vi "RL.vi"() -> ()   [LabVIEW 2019]
uses:
  <vilib>/Platform/TimedLoop/XDataNode/timing_clust.ctl
  <vilib>/Platform/TimedLoop/XDataNode/nitl_modes.ctl
  <vilib>/Platform/TimedLoop/XDataNode/wakeup.ctl
  <vilib>/Simulation/Shared/_Datatypes/SIM SISO Transfer Function.ctl
  <vilib>/myRIO/Instrument Drivers/Onboard IO/AI/typedefs/AI Reference.ctl
  <vilib>/myRIO/Common/Instrument Driver Framework/Utilities/typedefs/myRIO Generic Hardware Reference.ctl
  <vilib>/myRIO/Common/Instrument Driver Framework/Utilities/typedefs/Hardware Version Enum.ctl
  <vilib>/myRIO/Common/Instrument Driver Framework/Utilities/typedefs/myRIO v1.0 Reference.ctl
  <vilib>/myRIO/Common/Instrument Driver Framework/Utilities/typedefs/Generic FPGA Reference.ctl
  <vilib>/myRIO/Common/Instrument Driver Framework/myRIO v1.0/AI/typedefs/AI Channels List.ctl
  <vilib>/myRIO/Common/Instrument Driver Framework/myRIO v1.0/AI/typedefs/AI Channels Enum.ctl
  <vilib>/myRIO/Common/Instrument Driver Framework/Utilities/typedefs/Analog Scaling Constants List.ctl
  <vilib>/myRIO/Common/Instrument Driver Framework/Utilities/typedefs/Analog Scaling Constants.ctl
  <vilib>/userDefined/High Color/nirio_resource_hc.ctl
  <vilib>/Simulation/Shared/_Datatypes/SIM MIMO State Space.ctl
  <vilib>/myRIO/Instrument Drivers/Onboard IO/AO/typedefs/AO Reference.ctl
  <vilib>/myRIO/Common/Instrument Driver Framework/myRIO v1.0/AO/typedefs/AO Channels List.ctl
  <vilib>/myRIO/Common/Instrument Driver Framework/myRIO v1.0/AO/typedefs/AO Channels Enum.ctl
  <vilib>/myRIO/Common/Instrument Driver Framework/Utilities/vis/Is FPGA Ref Available.vi
  <vilib>/myRIO/Common/Instrument Driver Framework/myRIO v1.0/AI/vis/myRIO v1.1 Open AI.vi
  <vilib>/myRIO/Instrument Drivers/Onboard IO/AI/vis/Read.vi
  <vilib>/Simulation/DiscreteLinear/Implementation/NILVSim Discrete Transfer Function Direct.llb/SIM Discrete Transfer Function Diagram (SISO).vi
  <vilib>/Simulation/DiscreteLinear/Implementation/NILVSim Discrete State Space Direct.llb/SIM Discrete State Space Direct Diagram (SISO).vi
  <vilib>/myRIO/Common/Instrument Driver Framework/myRIO v1.0/AO/vis/myRIO v1.1 Open AO.vi
  <vilib>/myRIO/Instrument Drivers/Onboard IO/AO/vis/Write.vi
  <vilib>/myRIO/Common/Instrument Driver Framework/Utilities/vis/Validate Channels.vi
  <vilib>/myRIO/Common/Instrument Driver Framework/myRIO v1.0/AI/vis/myRIO v1.0 Reserve AI.vi
  <vilib>/Simulation/ContinuousLinear/Implementation/Shared/SIM Transfer Function Support.llb/SIM TransferFunction Normalize to Buffer.vi
  <vilib>/Simulation/DiscreteLinear/Implementation/Shared/SIM Init Discrete States.vi
  <vilib>/Simulation/DiscreteLinear/Implementation/NILVSim Discrete Transfer Function Direct.llb/SIM Transfer Function Direct core (SISO).vi
  <vilib>/Simulation/DiscreteLinear/Implementation/NILVSim Discrete State Space Direct.llb/NILVSim Discrete State Space Direct Diagram Core (SISO).vi
  <vilib>/myRIO/Common/Instrument Driver Framework/myRIO v1.0/AO/vis/myRIO v1.0 Reserve AO.vi
  <vilib>/myRIO/Common/Instrument Driver Framework/myRIO v1.0/AI/vis/myRIO v1.0 Build MUX Configuration AI.vi
  <vilib>/myRIO/Common/Instrument Driver Framework/myRIO v1.0/Resource Manager/vis/myRIO v1.0 Reserve Channel List.vi
  <vilib>/Simulation/ContinuousLinear/Implementation/Shared/SIM Transfer Function Support.llb/SIM TransferFunction Normalize.vi
  <vilib>/myRIO/Common/Instrument Driver Framework/myRIO v1.0/AO/vis/myRIO v1.0 Build MUX Configuration AO.vi
  <vilib>/myRIO/Common/Instrument Driver Framework/myRIO v1.0/Resource Manager/vis/myRIO v1.0 Reserve Channel.vi
  <vilib>/myRIO/Common/Instrument Driver Framework/myRIO v1.0/Resource Manager/vis/myRIO v1.0 Unreserve Channel.vi
  <vilib>/Simulation/Implementation/Shared/SIM Polynomials.llb/SIM Remove Zero Coefficients (DBL).vi
  <vilib>/myRIO/Common/Instrument Driver Framework/myRIO v1.0/Resource Manager/vis/myRIO v1.0 Build Mutex Name.vi
  <vilib>/Simulation/Implementation/Shared/SIM Polynomials.llb/SIM Divide Polynomials (DBL).vi
  <vilib>/Simulation/Implementation/Shared/SIM BuildSimErr.vi
  <vilib>/Utility/VariantDataType/GetNumericInfo.vi
  <vilib>/Utility/error.llb/Error Cluster From Error Code.vi
  <vilib>/myRIO/Common/Instrument Driver Framework/myRIO v1.0/myRIO v1.1 Open.vi
  <vilib>/myRIO/Common/Instrument Driver Framework/myRIO v1.0/AI/vis/myRIO v1.0 Get Scaling Constants AI.vi
  <vilib>/myRIO/Common/Instrument Driver Framework/Utilities/vis/IO Manager.vi
  <vilib>/myRIO/Common/Instrument Driver Framework/Utilities/vis/Configuration Manager.vi
  <vilib>/myRIO/Common/Instrument Driver Framework/myRIO v1.0/myRIO v1.0 Close.vi
  <vilib>/myRIO/Common/Instrument Driver Framework/myRIO v1.0/AI/vis/myRIO v1.0 Read AI.vi
  <vilib>/myRIO/Common/Instrument Driver Framework/myRIO v1.0/AO/vis/myRIO v1.0 Get Scaling Constants AO.vi
  <vilib>/myRIO/Common/Instrument Driver Framework/myRIO v1.0/AO/vis/myRIO v1.0 Write AO.vi
  <vilib>/platform/TimedLoop/XDataNode/XDataNode.xnode
  <vilib>/Simulation/Implementation/XNodeFramework/SimXNode/SimX.xnode
  <vilib>/myRIO/Express VI/Onboard IO/AI/AI Express VI.xnode
  <vilib>/myRIO/Instrument Drivers/Onboard IO/AI/vis/myRIO AI Open.xnode
  <vilib>/myRIO/Express VI/Onboard IO/AO/AO Express VI.xnode
  <vilib>/myRIO/Instrument Drivers/Onboard IO/AO/vis/myRIO AO Open.xnode
  <vilib>/Platform/TimedLoop/XDataNode/XDNodeRunTimeDep.lvlib
  <vilib>/myRIO/Instrument Drivers/Onboard IO/AI/AI.lvlib
  <vilib>/myRIO/Instrument Drivers/Onboard IO/AO/AO.lvlib
  <vilib>/ptbypt/NI_PtbyPt.lvlib
panel:
  in  "Chtter off":bool
  in  "psi":dbl=1.0
  in  "Ks":dbl=2.0
  in  "b":dbl=2.0
  in  "hm":dbl=0.01
  out "Current Output EM 2":dbl(graph)=0.21562841116112613
  in  "amplitude":dbl format="%0.2f"
  out "Impulse Pattern":dbl(graph)=9.575673587391975e-16
  in  "D":dbl=14.0
  in  "P":dbl=3000.0
  in  "stopNoise":bool=TRUE
  in  "gain_noise":dbl=200.0
  out "uniform white noise":dbl(graph)=-0.0005697152889172531
  in  "AmpWhitehNoise":dbl=1.0 format="%0.2f"
  out "Iteration Duration":i64(graph)=270
  in  "Max FRF current 0-1000mA":dbl=4.0
  in  "Stop FRF":bool=TRUE
  in  "esc":bool
  out "scope":T1(graph)={-45.41254239999998, -1.1831285746451028e-05, -0.0, "output y(k)"=9.575673587391975e-16, 544.5614125057525, "Numeric"=-3.431911784937208e-07, "Numeric"=9.18039926813991e-06}
  out "Current Output EM":dbl(graph)=0.04000924327853618
  in  "Stop EM + FRF":bool=TRUE
  out "left[V]":dbl=-0.0
  out "right[V]":dbl=-0.0
  out "um":dbl=414.0625424
  # "mA"
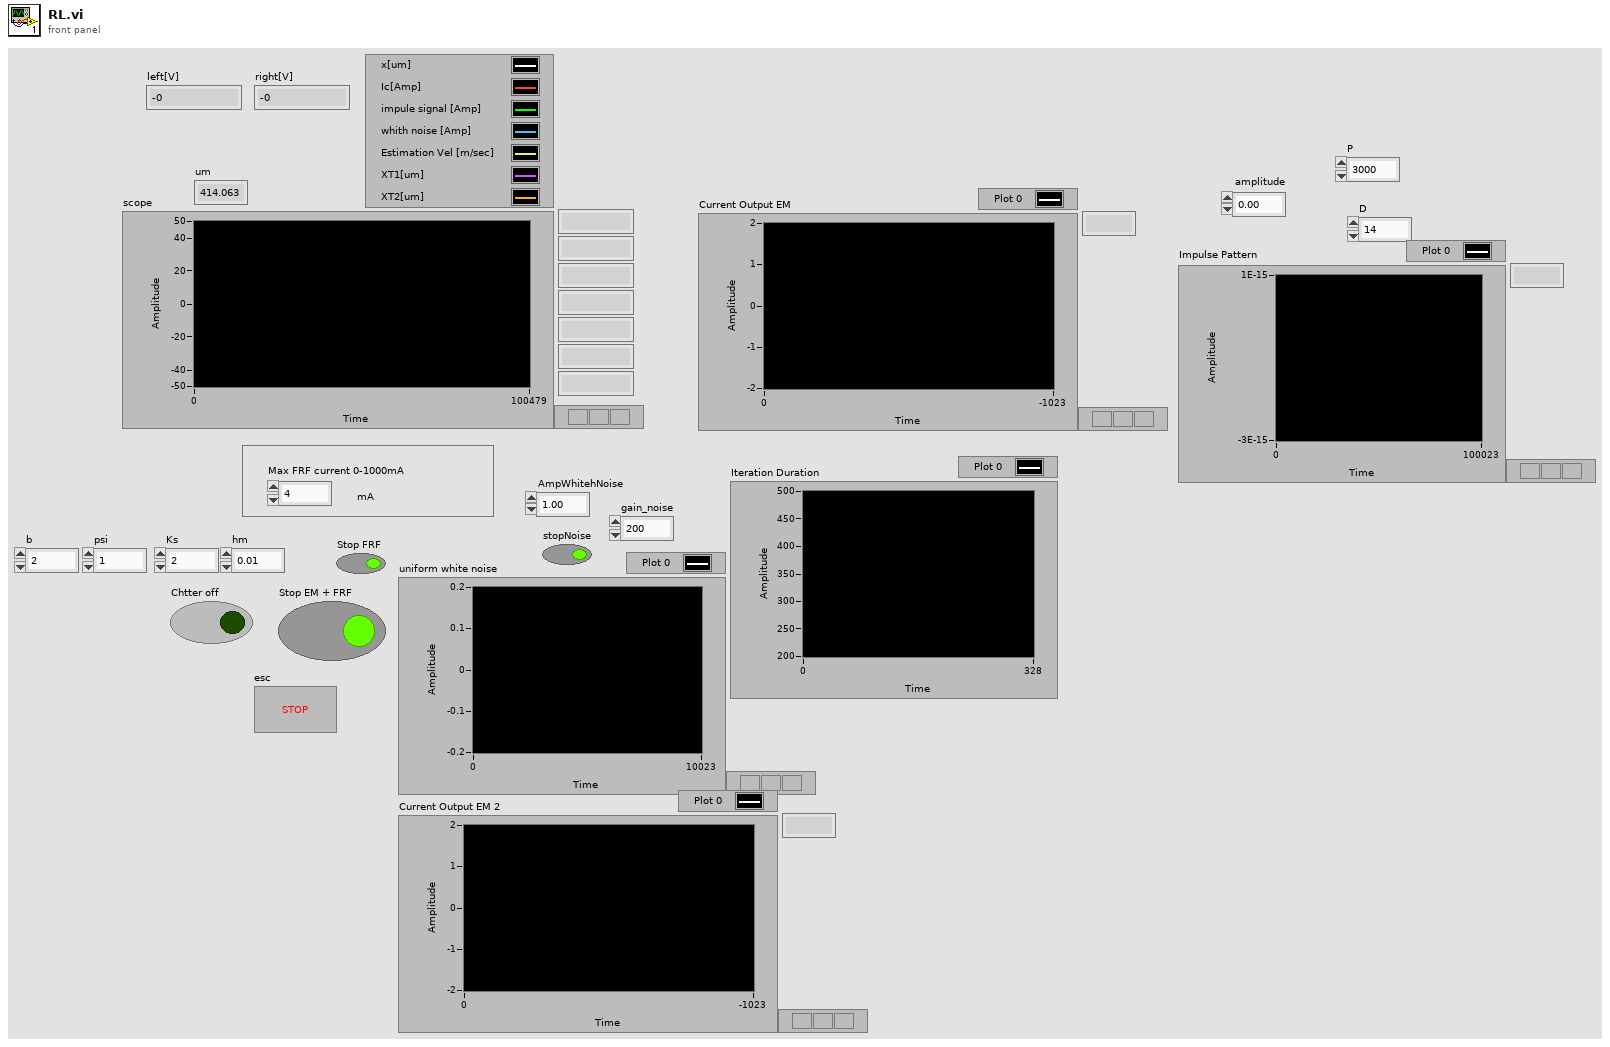
[diagram p1: front panel]
types:
  T1 = cluster{dbl, dbl, dbl, "output y(k)":dbl, dbl, "Numeric":dbl, "Numeric":dbl}
  T2 = typedef "XDNodeRunTimeDep.lvlib/timing_clust.ctl" = cluster{"Expected End [f-1]":u64, "Actual End [f-1]":u64, "Finished Late? [f-1]":bool, "Expected End [i-1]":u64, "Actual End [i-1]":u64, "Finished Late? [i-1]":bool, "Expected Start [i]":u64, "Actual Start [i]":u64, "Expected Start [f]":u64, "Actual Start [f]":u64, "Source Name":string, "Structure Name":string, "Period":i64, "Deadline":i64, "Offset":i64, "Start":i64, "Priority":i32, "Timeout":i32, "Mode":T3, "Wakeup Reason":T4, "Error":errorcluster, "Source Type":string, "Secondary Source Type":string, "Global End Time":u64, "Global Start Time":u64, "Frame Duration":u64, "Iteration Duration":u64, "Assigned CPU":i32, "I/O Scan Engine Mode":u32}
  T3 = typedef "XDNodeRunTimeDep.lvlib/nitl_modes.ctl" = enum32{"No Change", "Process missed periods, maintain original phase", "Discard missed periods, maintain original phase", "Process missed periods, ignore original phase", "Discard missed periods, ignore original phase"}
  T4 = typedef "XDNodeRunTimeDep.lvlib/wakeup.ctl" = enum32{"Normal", "Aborted", "Asynchronous wakeup", "Timing source error", "Timed loop error", "Timeout"}
  T5 = typedef "SIM MIMO State Space.ctl" = cluster{"A":dbl[][], "B":dbl[][], "C":dbl[][], "D":dbl[][]}
  T6 = typedef "SIM SISO Transfer Function.ctl" = cluster{"Numerator":dbl[], "Denominator":dbl[]}
  T7 = typedef "AI.lvlib/AI Reference.ctl" = cluster{"myRIO Reference":T8, "AI Channels List":T12, "AI Scaling Constants List":T14}
  T8 = typedef "myRIO Generic Hardware Reference.ctl" = cluster{"myRIO Model":T9, "myRIO Hardware Reference":T10}
  T9 = typedef "Hardware Version Enum.ctl" = enum16{"Unknown", "myRIO-1900", "myRIO-1950", "roboRIO", "NI ELVIS RIO CM", "ELVIS III"}
  T10 = typedef "myRIO v1.0 Reference.ctl" = cluster{"Generic FPGA Reference":T11, "Allow multiple opens":bool}
  T11 = typedef "Generic FPGA Reference.ctl" = refnum<k20>
  T12 = typedef "AI Channels List.ctl" = T13[]
  T13 = typedef "AI Channels Enum.ctl" = enum16{"Not Connected", "AudioIn/Left", "AudioIn/Right", "C/AI0", "C/AI1", "A/AI0", "A/AI1", "A/AI2", "A/AI3", "A/AI4", "A/AI5", "A/AI6", "A/AI7", "B/AI0", "B/AI1", "B/AI2", "B/AI3", "B/AI4", "B/AI5", "B/AI6", "B/AI7", "AI/AI0", "AI/AI1", "AI/AI2", "AI/AI3", "A/AI0 (DIFF)", "A/AI1 (DIFF)", "A/AI2 (DIFF)", "A/AI3 (DIFF)", "B/AI0 (DIFF)", "B/AI1 (DIFF)", "B/AI2 (DIFF)", "B/AI3 (DIFF)"}
  T14 = typedef "Analog Scaling Constants List.ctl" = T15[]
  T15 = typedef "Analog Scaling Constants.ctl" = cluster{"LSB Weight (Volts)":dbl, "Offset (Volts)":dbl, "Signed?":bool}
  T16 = typedef "nirio_resource_hc.ctl" = tag
  T17 = typedef "AO.lvlib/AO Reference.ctl" = cluster{"myRIO Reference":T8, "AO Channel List":T18, "AO Scaling Constant List":T14}
  T18 = typedef "AO Channels List.ctl" = T19[]
  T19 = typedef "AO Channels Enum.ctl" = enum16{"Not Connected", "AudioOut/Left", "AudioOut/Right", "C/AO0", "C/AO1", "A/AO0", "A/AO1", "B/AO0", "B/AO1"}
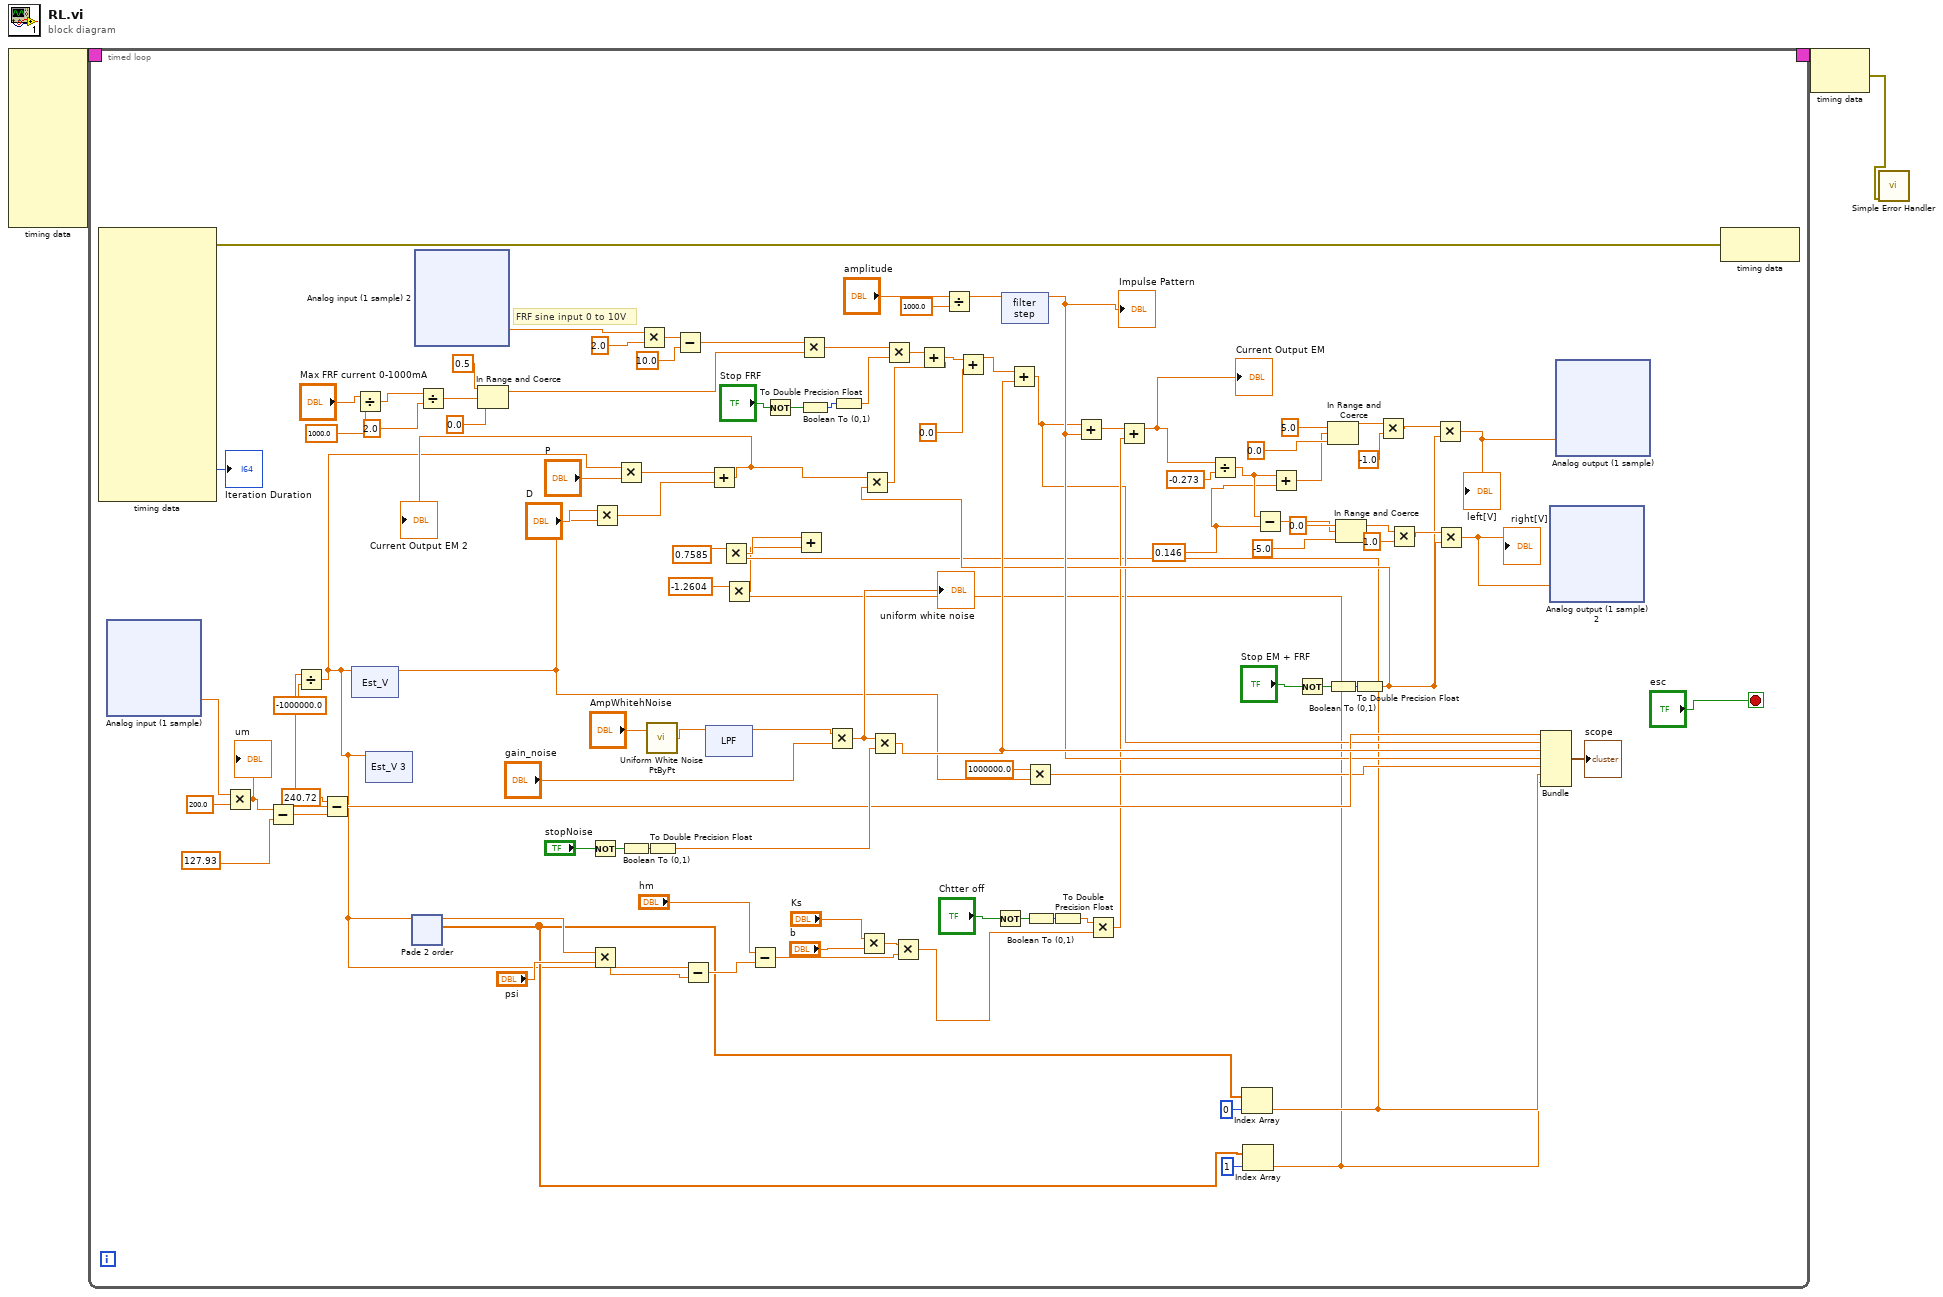
[diagram p0: block diagram]
diagram:
  n1 = node-c288() -> (w3:T2)  [unwired: 10 in]
  n2 = timed-loop {
    timing: w3 -> [_]
    timing-out: [_] -> w2
    stop <- "esc" stop-if-true
    w68 = 0.146 ("y")
    # "FRF sine input 0 to 10V"
    n3 = node-c288() -> (w109:errorcluster, →"Iteration Duration":i64)  [unwired: 1 in, 15 out]
    n4 = xnode "Analog input (1 sample)"() -> ("C/AI1 (AI1)"=w65:dbl)  [unwired: 1 in, 1 out]
    n5 = Multiply(x=w65, y=200.0) -> (x*y=w107:dbl)
    "um" <- w107
    n6 = Subtract(x=w107, y=127.93) -> (x-y=w106:dbl)
    n7 = Subtract(x=240.72, y=w106) -> (x-y=w48:dbl)
    n8 = Divide(x=w48, y=-1000000.0) -> (x/y=w14:dbl)
    n9 = xnode "Est_V"("input u(k)"=w14) -> ("output y(k)"=w5:dbl)  [unwired: 2 in, 1 out]
    n10 = Divide(x="Max FRF current 0-1000mA", y=1000.0) -> (x/y=w75:dbl)
    n11 = xnode "Est_V 3"("input u(k)"=w14) -> ()  [unwired: 2 in, 2 out]
    n12 = xnode "Pade 2 order"("input u(k)"=w14) -> ("state x(k+1)"=w17:dbl[], "output y(k)"=w18:dbl)  [unwired: 2 in, 2 out]
    n13 = xnode "Analog input (1 sample) 2"() -> ("C/AI0 (AI0)"=w86:dbl)  [unwired: 1 in, 1 out]
    n14 = Divide(x=w75, y=2.0) -> (x/y=w79:dbl)
    n15 = In Range and Coerce(upper limit=0.5, x=w79, lower limit=0.0) -> (coerced(x)=w76:dbl)  [unwired: 1 out]
    n16 = Not(x="stopNoise") -> (.not. x?=w56:bool)
    n17 = Multiply(x=w18, y="psi") -> (x*y=w21:dbl)
    n18 = Multiply(x="D", y=w5) -> (x*y=w46:dbl)
    n19 = Multiply(x=w14, y="P") -> (x*y=w47:dbl)
    n20 = Boolean To (0,1)(Boolean=w56) -> (0, 1=w57:i16)
    n21 = Multiply(x=w86, y=2.0) -> (x*y=w84:dbl)
    n22 = call <vilib>:"Uniform White Noise PtByPt.vi"("amplitude"="AmpWhitehNoise") -> ("uniform white noise"=w58:dbl)  [unwired: 2 in]
    n23 = To Double Precision Float(number=w57) -> (double precision float=w52:dbl)
    n24 = Subtract(x=w84, y=10.0) -> (x-y=w81:dbl)
    n25 = Subtract(x=w14, y=w21) -> (x-y=w20:dbl)
    n26 = xnode "LPF"("input u(k)"=w58) -> ("output y(k)"=w55:dbl)  [unwired: 2 in, 1 out]
    n27 = Add(x=w47, y=w46) -> (x+y=w34:dbl)
    "Current Output EM 2" <- w34
    n28 = Subtract(x="hm", y=w20) -> (x-y=w32:dbl)
    n29 = Not(x="Stop FRF") -> (.not. x?=w89:bool)
    n30 = Multiply(x=w81, y=w76) -> (x*y=w82:dbl)
    n31 = Boolean To (0,1)(Boolean=w89) -> (0, 1=w88:i16)
    n32 = Multiply(x=w55, y="gain_noise") -> (x*y=w51:dbl)
    "uniform white noise" <- w51
    n33 = To Double Precision Float(number=w88) -> (double precision float=w87:dbl)
    n34 = Multiply(x="Ks", y="b") -> (x*y=w33:dbl)
    n35 = Multiply(x=w51, y=w52) -> (x*y=w50:dbl)
    n36 = Multiply(x=w82, y=w87) -> (x*y=w91:dbl)
    n37 = Multiply(x=w33, y=w32) -> (x*y=w24:dbl)
    n38 = Divide(x="amplitude", y=1000.0) -> (x/y=w42:dbl)
    n39 = Not(x="Chtter off") -> (.not. x?=w26:bool)
    n40 = xnode "filter step"("input u(k)"=w42) -> ("output y(k)"=w39:dbl)  [unwired: 2 in, 1 out]
    "Impulse Pattern" <- w39
    n41 = Multiply(x=1000000.0, y=w5) -> (x*y=w38:dbl)
    n42 = Boolean To (0,1)(Boolean=w26) -> (0, 1=w27:i16)
    n43 = To Double Precision Float(number=w27) -> (double precision float=w25:dbl)
    n44 = Multiply(x=w25, y=w24) -> (x*y=w15:dbl)
    n45 = Index Array(array=w17, index=0 ("index (row)")) -> (element=w12:dbl)
    n46 = Multiply(x=0.7585, y=w12) -> (x*y=w8:dbl)
    n47 = Index Array(array=w17, index=1) -> (element=w11:dbl)
    n48 = Multiply(x=-1.2604, y=w11) -> (x*y=w7:dbl)
    n49 = Add(x=w8, y=w7) -> ()  [unwired: 1 out]
    n50 = Not(x="Stop EM + FRF") -> (.not. x?=w94:bool)
    n51 = Boolean To (0,1)(Boolean=w94) -> (0, 1=w96:i16)
    n52 = To Double Precision Float(number=w96) -> (double precision float=w35:dbl)
    n53 = Multiply(x=w34, y=w35) -> (x*y=w36:dbl)
    n54 = Add(x=w91, y=w36) -> (x+y=w49:dbl)
    n55 = Add(x=w49, y=0.0) -> (x+y=w6:dbl)
    n56 = Add(x=w6, y=w50) -> (x+y=w13:dbl)
    n57 = Add(x=w13, y=w39) -> (x+y=w40:dbl)
    n58 = Add(x=w40, y=w15) -> (x+y=w16:dbl)
    "Current Output EM" <- w16
    n59 = Divide(x=w16, y=-0.273) -> (x/y=w69:dbl)
    n60 = Subtract(x=w69, y=w68) -> (x-y=w70:dbl)
    n61 = Add(x=w69, y=w68) -> (x+y=w71:dbl)
    n62 = In Range and Coerce(upper limit=5.0 ("x"), x=w71, lower limit=0.0) -> (coerced(x)=w62:dbl)  [unwired: 1 out]
    n63 = In Range and Coerce(upper limit=0.0 ("x"), x=w70, lower limit=-5.0) -> (coerced(x)=w99:dbl)  [unwired: 1 out]
    n64 = Multiply(x=w62, y=-1.0) -> (x*y=w67:dbl)
    n65 = Multiply(x=w99, y=1.0) -> (x*y=w66:dbl)
    n66 = Multiply(x=w67, y=w35) -> (x*y=w64:dbl)
    "left[V]" <- w64
    n67 = Multiply(x=w66, y=w35) -> (x*y=w63:dbl)
    "right[V]" <- w63
    n68 = Bundle(w48, w13, w50, "output y(k)"=w39, w38, "Numeric"=w12, "Numeric"=w11) -> (→"scope":T1)  [unwired: 1 in]
    n69 = xnode "Analog output (1 sample) 2"("C/AO1 (AO1)"=w63) -> ()  [unwired: 1 in, 1 out]
    n70 = xnode "Analog output (1 sample)"("C/AO0 (AO0)"=w64) -> ()  [unwired: 1 in, 1 out]
    n71 = node-c288(w109) -> ()  [unwired: 1 out]
  }
  n72 = node-c288(w2) -> (w1:errorcluster)
  n73 = call <vilib>:"Simple Error Handler.vi"("error in (no error)"=w1) -> ()  [unwired: 4 in, 5 out]
